vi "DT_Find Next Triangulation_Base Point_Init.vi"(7 "left/right pt (right:F)":bool, 8 "search point":i32, 9 "external point":i32, 10 "Triangles In":i32[][](array[numeric]), 11 "Points In":cluster{"x":dbl, "y":dbl, "index":i32}[](array[cluster])) -> (0 "done?":bool, 1 "global idx":i32, 2 "local idx":i32, 3 "triangle":i32)   [LabVIEW 2017, in "NI_AAL_Geometry.lvlib"]
uses:
  <vilib>/Analysis/NI_AAL_Geometry.lvlib
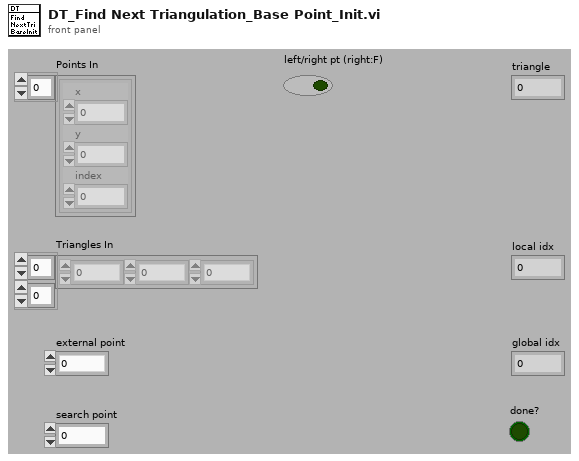
[diagram p1: front panel]
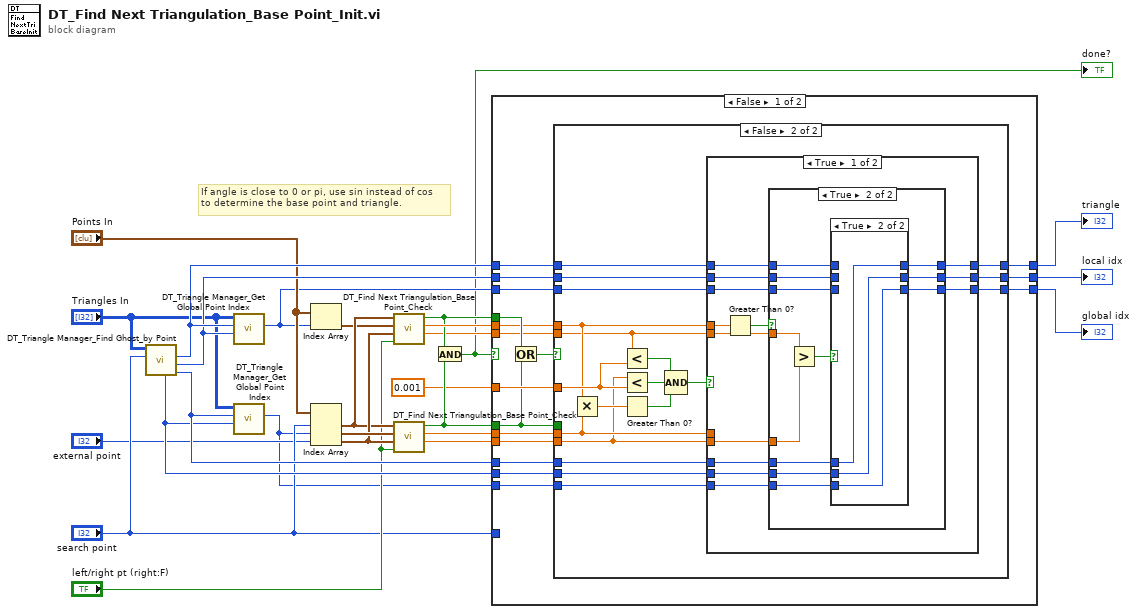
[diagram p0: block diagram]
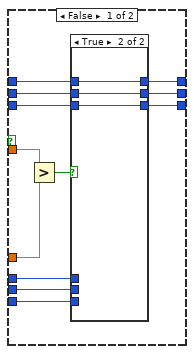
[diagram p4: hidden frame]
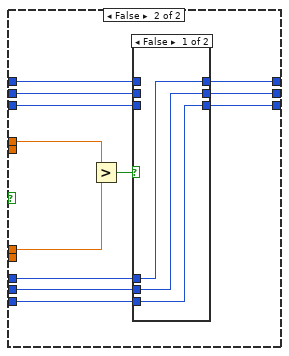
[diagram p7: hidden frame]
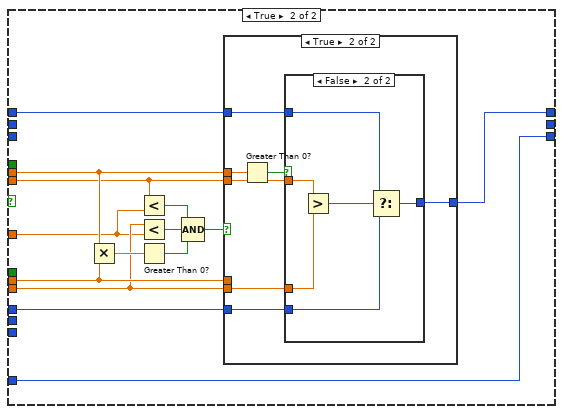
[diagram p9: hidden frame]
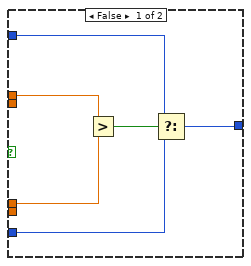
[diagram p10: hidden frame]
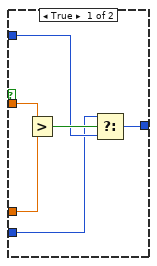
[diagram p11: hidden frame]
diagram:
  # "If angle is close to 0 or pi, use sin instead of cos\nto determine the base point and triangle."
  n1 = call <vilib>:"DT_Triangle Manager_Find Ghost_by Point.vi"("point"="search point", "Triangles"="Triangles In") -> ("triangle 2"=w24:i32, "point idx 1"=w25:i32, "triangle 1"=w26:i32, "point idx 2"=w23:i32)  [unwired: 6 out]
  n2 = call <vilib>:"DT_Triangle Manager_Get Global Point Index.vi"("local idx"=w25, "triangle"=w26, "Triangles"="Triangles In") -> ("global idx"=w8:i32)  [unwired: 8 out]
  n3 = call <vilib>:"DT_Triangle Manager_Get Global Point Index.vi"("local idx"=w23, "triangle"=w24, "Triangles"="Triangles In") -> ("global idx"=w9:i32)  [unwired: 8 out]
  n4 = Index Array(array="Points In", index=w8) -> (element=w15:cluster{"x":dbl, "y":dbl, "index":i32})
  n5 = Index Array(array="Points In", index #1="search point", index #2=w9, index #3="external point") -> (element #1=w16:cluster{"x":dbl, "y":dbl, "index":i32}, element #2=w22:cluster{"x":dbl, "y":dbl, "index":i32}, element #3=w17:cluster{"x":dbl, "y":dbl, "index":i32})
  n6 = call <vilib>:"DT_Find Next Triangulation_Base Point_Check.vi"("left/right pt (right:F)"="left/right pt (right:F)", "p 3"=w17, "p 2"=w15, "p 1"=w16) -> ("sin"=w6:dbl, "cos"=w19:dbl, "pass?"=w18:bool)  [unwired: 5 out]
  n7 = call <vilib>:"DT_Find Next Triangulation_Base Point_Check.vi"("left/right pt (right:F)"="left/right pt (right:F)", "p 3"=w17, "p 2"=w22, "p 1"=w16) -> ("sin"=w5:dbl, "cos"=w20:dbl, "pass?"=w21:bool)  [unwired: 5 out]
  n8 = And(x=w18, y=w21) -> (x .and. y?=w4:bool)
  "done?" <- w4
  n9 = case shown="False" w4 {
    tunnel: w19 -> [w34 w152]
    tunnel: w20 -> [w32 w151]
    tunnel: w26 -> [w42 w159]
    tunnel: w24 -> [w41 w158]
    tunnel: "search point" -> [_ w146]
    tunnel: [w30 w157] -> w13
    tunnel: w21 -> [w27 _]
    tunnel: w18 -> [w43 _]
    tunnel: w25 -> [w40 _]
    tunnel: w23 -> [w39 _]
    tunnel: w8 -> [w38 _]
    tunnel: w9 -> [w37 _]
    tunnel: w6 -> [w35 w149]
    tunnel: w5 -> [w33 w148]
    tunnel: 0.001 ("y") -> [w36 w147]
    tunnel: [w29 w146] -> w2
    tunnel: [w28 _] -> w1
    frame False {
      n10 = Or(x=w43, y=w27) -> (x .or. y?=w31:bool)
      n11 = case shown="False" w31 {
        tunnel: w42 -> [w53 w78]
        tunnel: w41 -> [w52 w77]
        tunnel: w40 -> [w51 w76]
        tunnel: w39 -> [w50 w75]
        tunnel: w38 -> [w49 w74]
        tunnel: w37 -> [w48 w73]
        tunnel: w36 -> [_ w68]
        tunnel: w35 -> [_ w61]
        tunnel: w34 -> [_ w67]
        tunnel: w33 -> [_ w60]
        tunnel: w32 -> [_ w66]
        tunnel: [w47 w64] -> w30
        tunnel: [w46 w62] -> w29
        tunnel: [w45 w63] -> w28
        tunnel: w27 -> [w44 _]
        frame True {
          n12 = case shown="False" w44 {
            tunnel: w53 -> [_ w59]
            tunnel: w52 -> [w56 _]
            tunnel: w51 -> [_ w58]
            tunnel: w50 -> [w55 _]
            tunnel: [w56 w59] -> w47
            tunnel: [w55 w58] -> w45
            tunnel: w49 -> [_ w57]
            tunnel: w48 -> [w54 _]
            tunnel: [w54 w57] -> w46
            frame False {
            }
            frame True {
            }
          }
        }
        frame False {
          n13 = Multiply(x=w67, y=w66) -> (x*y=w70:dbl)
          n14 = Less?(x=w61, y=w68) -> (x < y?=w72:bool)
          n15 = Less?(x=w60, y=w68) -> (x < y?=w71:bool)
          n16 = Greater Than 0?(x=w70) -> (x > 0?=w69:bool)
          n17 = Compound Arithmetic op=AND(w72, w71, w69) -> (w65:bool)
          n18 = case shown="True" w65 {
            tunnel: w78 -> [w91 w139]
            tunnel: w77 -> [w90 w138]
            tunnel: w76 -> [w89 w137]
            tunnel: w75 -> [w88 w136]
            tunnel: w74 -> [w87 w135]
            tunnel: w73 -> [w86 w134]
            tunnel: w67 -> [w83 w133]
            tunnel: w66 -> [_ w132]
            tunnel: [w81 w130] -> w64
            tunnel: [w80 w129] -> w63
            tunnel: [w79 w128] -> w62
            tunnel: w61 -> [w85 _]
            tunnel: w60 -> [w84 _]
            frame True {
              n19 = Greater Than 0?(x=w83) -> (x > 0?=w82:bool)
              n20 = case shown="True" w82 {
                tunnel: w91 -> [w100 w118]
                tunnel: w90 -> [w94 w112]
                tunnel: [w99 w117] -> w81
                tunnel: w89 -> [w98 w116]
                tunnel: w88 -> [w93 w111]
                tunnel: w85 -> [w103 w121]
                tunnel: w84 -> [w102 w120]
                tunnel: [w97 w115] -> w80
                tunnel: w87 -> [w96 w114]
                tunnel: w86 -> [w92 w110]
                tunnel: [w95 w113] -> w79
                frame False {
                  n21 = Greater?(x=w103, y=w102) -> (0:w101:bool)
                  n22 = case shown="True" w101 {
                    tunnel: w100 -> [_ w109]
                    tunnel: [w106 w109] -> w99
                    tunnel: w98 -> [_ w108]
                    tunnel: [w105 w108] -> w97
                    tunnel: w96 -> [_ w107]
                    tunnel: [w104 w107] -> w95
                    tunnel: w94 -> [w106 _]
                    tunnel: w93 -> [w105 _]
                    tunnel: w92 -> [w104 _]
                    frame False {
                    }
                    frame True {
                    }
                  }
                }
                frame True {
                  n23 = Greater?(x=w121, y=w120) -> (0:w119:bool)
                  n24 = case shown="True" w119 {
                    tunnel: w118 -> [w124 _]
                    tunnel: [w124 w127] -> w117
                    tunnel: w116 -> [w123 _]
                    tunnel: [w123 w126] -> w115
                    tunnel: w114 -> [w122 _]
                    tunnel: [w122 w125] -> w113
                    tunnel: w112 -> [_ w127]
                    tunnel: w111 -> [_ w126]
                    tunnel: w110 -> [_ w125]
                    frame False {
                    }
                    frame True {
                    }
                  }
                }
              }
            }
            frame False {
              n25 = Greater?(x=w133, y=w132) -> (0:w131:bool)
              n26 = case shown="False" w131 {
                tunnel: w139 -> [_ w145]
                tunnel: [w142 w145] -> w130
                tunnel: w137 -> [_ w144]
                tunnel: [w141 w144] -> w129
                tunnel: w135 -> [_ w143]
                tunnel: [w140 w143] -> w128
                tunnel: w138 -> [w142 _]
                tunnel: w136 -> [w141 _]
                tunnel: w134 -> [w140 _]
                frame False {
                }
                frame True {
                }
              }
            }
          }
        }
      }
    }
    frame True {
      n27 = Multiply(x=w152, y=w151) -> (x*y=w154:dbl)
      n28 = Less?(x=w149, y=w147) -> (x < y?=w156:bool)
      n29 = Less?(x=w148, y=w147) -> (x < y?=w155:bool)
      n30 = Greater Than 0?(x=w154) -> (x > 0?=w153:bool)
      n31 = Compound Arithmetic op=AND(w156, w155, w153) -> (w150:bool)
      n32 = case shown="True" w150 {
        tunnel: w159 -> [w164 w172]
        tunnel: w158 -> [w163 w171]
        tunnel: [w162 w170] -> w157
        tunnel: w152 -> [w161 w168]
        tunnel: w151 -> [w160 _]
        tunnel: w149 -> [_ w169]
        tunnel: w148 -> [_ w166]
        frame False {
          n33 = Greater?(x=w161, y=w160) -> (0:w165:bool)
          n34 = Select(t=w164, s=w165, f=w163) -> (s? t:f=w162:i32)
        }
        frame True {
          n35 = Greater Than 0?(x=w168) -> (x > 0?=w167:bool)
          n36 = case shown="False" w167 {
            tunnel: w172 -> [w174 w183]
            tunnel: w171 -> [w173 w182]
            tunnel: [w177 w181] -> w170
            tunnel: w166 -> [w176 w180]
            tunnel: w169 -> [w175 w179]
            frame True {
              n37 = Greater?(x=w175, y=w176) -> (0:w178:bool)
              n38 = Select(t=w173, s=w178, f=w174) -> (s? t:f=w177:i32)
            }
            frame False {
              n39 = Greater?(x=w179, y=w180) -> (0:w184:bool)
              n40 = Select(t=w183, s=w184, f=w182) -> (s? t:f=w181:i32)
            }
          }
        }
      }
    }
  }
  "triangle" <- w13
  "global idx" <- w2
  "local idx" <- w1
